vi "Check Number In Lower E-Series.vi"(9 "1D sel":T1, 10 "2D sel":T1, 11 "E Serie":u16[](array[numeric])) -> (3 "In Serie?":bool)   [LabVIEW 2018]
uses:
  digit--enum.ctl
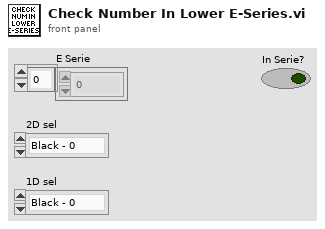
[diagram p1: front panel]
types:
  T1 = typedef "digit--enum.ctl" = enum16{"Black - 0", "Brown - 1", "Red - 2", "Orange - 3", "Yellow - 4", "Green - 5", "Blue - 6", "Violet - 7", "Grey - 8", "White - 9"}
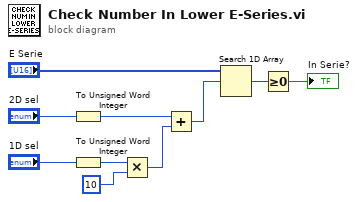
[diagram p0: block diagram]
diagram:
  n1 = To Unsigned Word Integer(number="2D sel") -> (unsigned 16bit integer=w5:u16)
  n2 = To Unsigned Word Integer(number="1D sel") -> (unsigned 16bit integer=w3:u16)
  n3 = Multiply(x=w3, y=u16 10) -> (x*y=w6:u16)
  n4 = Add(x=w5, y=w6) -> (x+y=w8:u16)
  n5 = Search 1D Array(1D array="E Serie", element=w8) -> (index of element=w9:i32)  [unwired: 1 in]
  n6 = Greater Or Equal To 0?(x=w9) -> (x >= 0?=→"In Serie?":bool)
